vi "New RegRead Command.vi"(0 "RFFE RegRead Command in":refnum<class "RFFE RegRead Command.lvclass">, 1 "Alias":string, 5 "Slave Address":T2=12 format="%02x", 7 "Register Address":T1 format="%02x", 11 "error in (no error)":errorcluster) -> (4 "RFFE RegRead Command out":refnum<class "RFFE RegRead Command.lvclass">, 15 "error out":errorcluster)   [LabVIEW 2018, in "MIPI RFFE API.lvlib" / "RFFE RegRead Command.lvclass"]
uses:
  RFFE RegRead Command.lvclass
  C:/Users/semoore/Projects/mipi-rffe-labview-oop/Standard Command/RFFE Standard Command.lvclass
  Slave Address.ctl
  Register Address.ctl
  Register Data.ctl
  Standard Command/RFFE Standard Command.lvclass
  MIPI RFFE API.lvlib
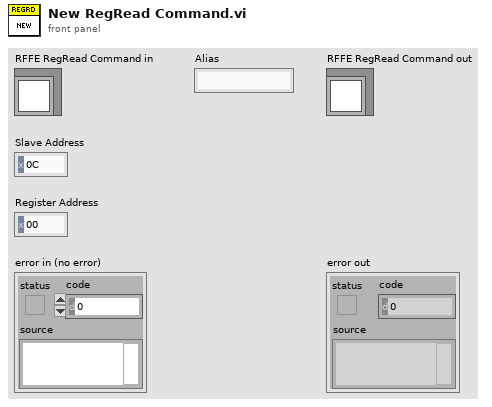
[diagram p1: front panel]
types:
  T1 = typedef "MIPI RFFE API.lvlib/Register Address.ctl" = u16
  T2 = typedef "MIPI RFFE API.lvlib/Slave Address.ctl" = u8
  T3 = typedef "MIPI RFFE API.lvlib/Register Data.ctl" = u8
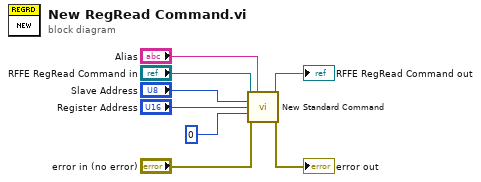
[diagram p0: block diagram]
diagram:
  n1 = call "New Standard Command.vi"("RFFE Standard Command in"="RFFE RegRead Command in", "Alias"="Alias", "Slave Address"="Slave Address", "Register Address"="Register Address", "Register Data"=T3 0, "error in (no error)"="error in (no error)") -> ("RFFE Standard Command out"=→"RFFE RegRead Command out":refnum<class "RFFE RegRead Command.lvclass">, "error out"=→"error out":errorcluster)  [unwired: 8 in]
